vi "Call Open VI.vi"(8 "error in (no error)":errorcluster, 11 "Refnum in":refnum<k21>) -> (0 "error out":errorcluster, 3 "nismPluginAxisBaseClass out":refnum<class "nismPluginAxisBaseClass.lvclass">)   [LabVIEW 2014]
uses:
  <vilib>/Motion/plugins/PluginFramework/nismPluginAxisBase/nismPluginAxisBaseClass.lvclass
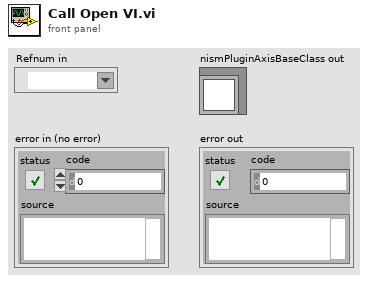
[diagram p1: front panel]
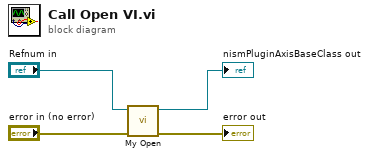
[diagram p0: block diagram]
diagram:
  n1 = call "My Open.vi"("error in (no error)"="error in (no error)", "Axis"="Refnum in") -> ("error out"=→"error out":errorcluster, "Base Axis Out"=→"nismPluginAxisBaseClass out":refnum<class "nismPluginAxisBaseClass.lvclass">)  [unwired: 8 in]
